vi "onTestExecution.vi"(7 "Name":string, 8 "error in (no error)":errorcluster, 11 "Test Runner.Collection in":refnum<class "Test Runner.Collection.lvclass">) -> (0 "error out":errorcluster, 3 "Test Runner.Collection out":refnum<class "Test Runner.Collection.lvclass">)   [LabVIEW 2013, in "Caraya.lvlib" / "Test Runner.Collection.lvclass"]
uses:
  Test Runner.Collection.lvclass
  Test Runner.Collection.lvclass/Test Runner.Collection.ctl
  Test Runner/Test Runner.lvclass
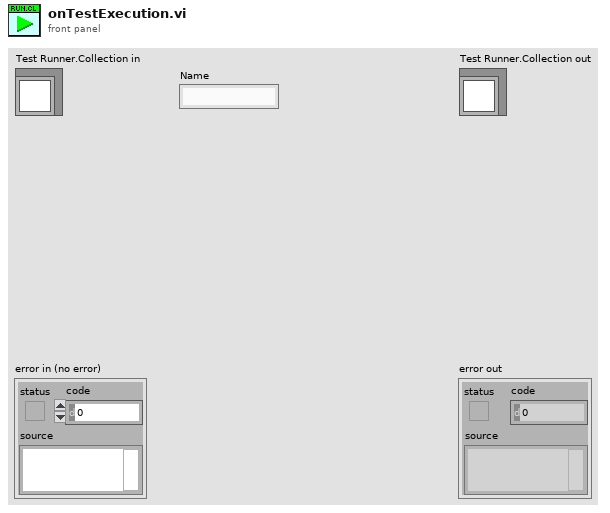
[diagram p1: front panel]
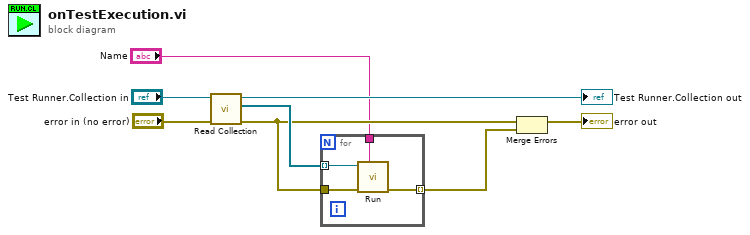
[diagram p0: block diagram]
diagram:
  n1 = call "Read Collection.vi"("error in (no error)"="error in (no error)", "Test Runner.Collection in"="Test Runner.Collection in") -> ("error out"=w3:errorcluster, "Test Runners"=w7:refnum<class "Test Runner.lvclass">[], "Test Runner.Collection out"=→"Test Runner.Collection out":refnum<class "Test Runner.Collection.lvclass">)  [unwired: 7 in]
  n2 = for {
    tunnel: w7 -> [w12] mode=indexing
    tunnel: w3 -> [w11]
    tunnel: [w10] -> w8 mode=indexing
    tunnel: "Name" -> [w9]
    n3 = call "Run.vi"("Name"=w9, "error in (no error)"=w11, "Test Runner in"=w12) -> ("error out"=w10:errorcluster)  [unwired: 7 in, 1 out]
  }
  n4 = Merge Errors(w3, w8) -> (→"error out":errorcluster)
